vi "ALARM Check DC.vi"(8 "error in (no error)":errorcluster, 9 "Motion Status":bool=TRUE, 10 "SP":dbl[](array[numeric]), 11 "register values":dbl[](array[numeric])) -> (0 "error out":errorcluster, 3 "Array":u32[](array[numeric]))   [LabVIEW 2020, in "QCT ALARM.lvlib"]
uses:
  QCT ALARM.lvlib
  support/PCT FGV CMD.ctl
panel:
  out "Waveform Graph":dbl[](graph)
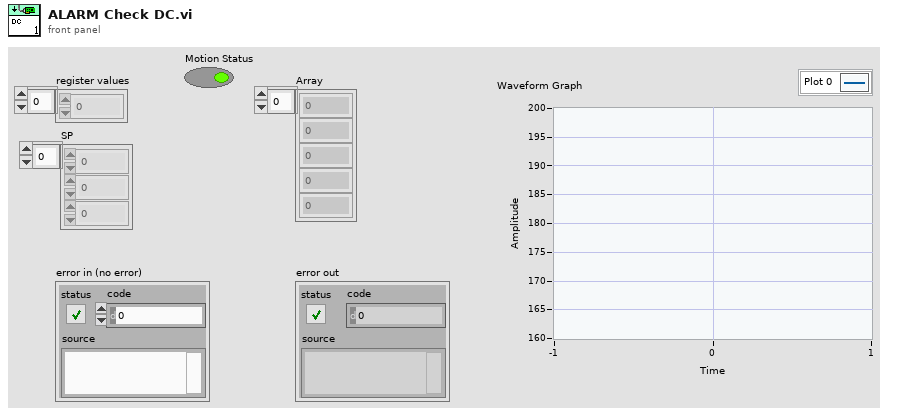
[diagram p1: front panel]
types:
  T1 = typedef "PCT FGV CMD.ctl" = enum16{"INIT", "GET", "SET"}
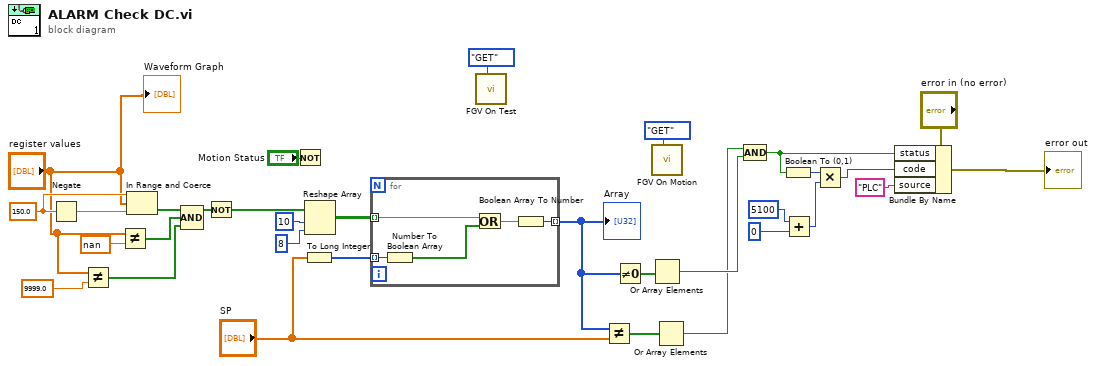
[diagram p0: block diagram]
diagram:
  w26 = 150.0 ("Threshold")
  n1 = Negate(x=w26) -> (-x=w25:dbl)
  n2 = Not Equal?(x="register values", y=9999.0 ("Threshold")) -> (x != y?=w1:bool[])
  n3 = Not Equal?(x="register values", y=nan ("Threshold")) -> (x != y?=w14:bool[])
  n4 = In Range and Coerce(upper limit=w26, x="register values", lower limit=w25) -> (In Range?=w30:bool[])  [unwired: 1 out]
  n5 = Compound Arithmetic op=AND(w30, w14, w1) -> (w15:bool[])
  n6 = Not(x=w15) -> (.not. x?=w32:bool[])
  n7 = Not(x="Motion Status") -> ()  [unwired: 1 out]
  n8 = To Long Integer(number="SP") -> (32bit integer=w12:i32[])
  n9 = Reshape Array(w32, 10 ("dimension size"), 8 ("dimension size")) -> (w29:bool[][])
  n10 = for {
    tunnel: [w37] -> w11 mode=indexing
    tunnel: w29 -> [w36] mode=indexing
    tunnel: w12 -> [w35] mode=indexing
    n11 = Number To Boolean Array(number=w35) -> (Boolean array=w33:bool[])
    n12 = Or(x=w36, y=w33) -> (x .or. y?=w34:bool[])
    n13 = Boolean Array To Number(Boolean array=w34) -> (number=w37:u32)
  }
  "Array" <- w11
  n14 = call "FGV On Test.vi"("CMD"=PCT_FGV_CMD."GET") -> ()  [unwired: 9 in, 2 out]
  n15 = Not Equal?(x=w11, y="SP") -> (x != y?=w31:bool[])
  n16 = Not Equal To 0?(x=w11) -> (x != 0?=w10:bool[])
  n17 = call "FGV On Motion.vi"("CMD"=PCT_FGV_CMD."GET") -> ()  [unwired: 9 in, 2 out]
  n18 = Or Array Elements(Boolean array=w10) -> (logical OR=w6:bool)
  n19 = Or Array Elements(Boolean array=w31) -> (logical OR=w5:bool)
  n20 = Compound Arithmetic op=AND(w5, w6) -> (w4:bool)
  n21 = Boolean To (0,1)(Boolean=w4) -> (0, 1=w23:i16)
  n22 = Add(x=5100 ("code"), y=0) -> (x+y=w21:i32)
  n23 = Multiply(x=w23, y=w21) -> (x*y=w22:i32)
  n24 = Bundle By Name(cluster="error in (no error)", "status"=w4, "code"=w22, "source"="PLC") -> (→"error out":errorcluster)
  "Waveform Graph" <- "register values"
